vi "Best_Match.vi"(2 "Input String":string, 3 "String Options":string[](array[string])) -> (0 "Good Match":bool, 1 "index of element":i32)   [LabVIEW 2018]
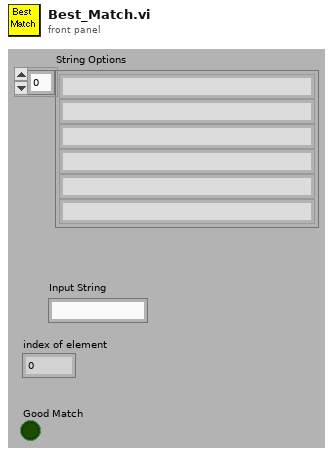
[diagram p1: front panel]
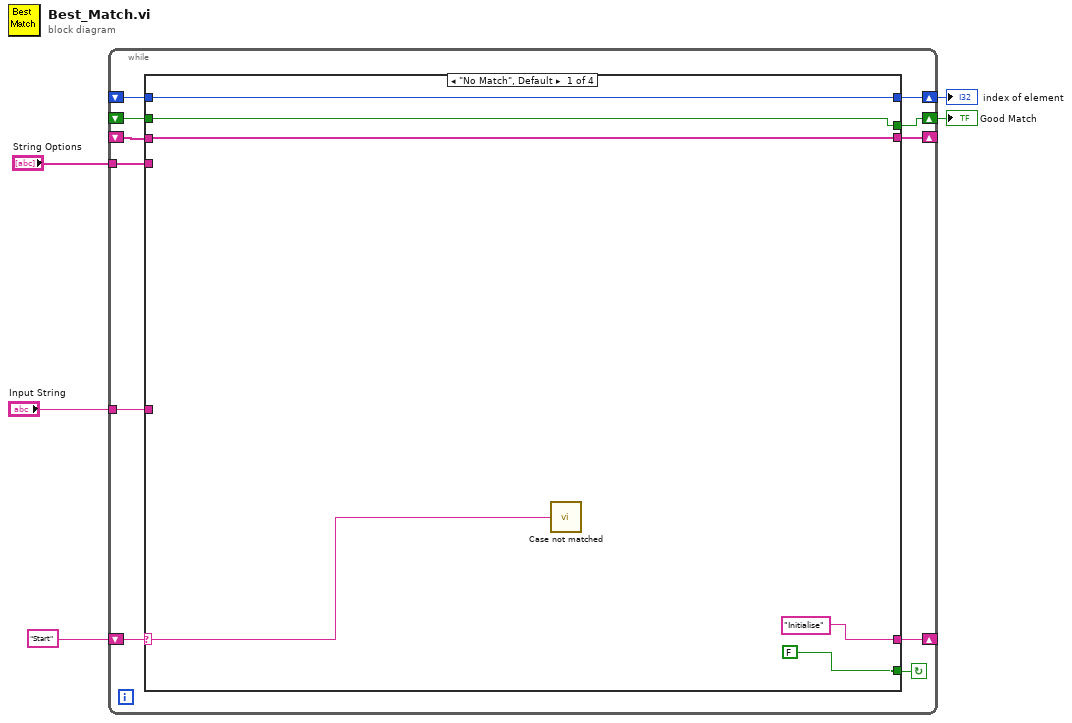
[diagram p0: block diagram]
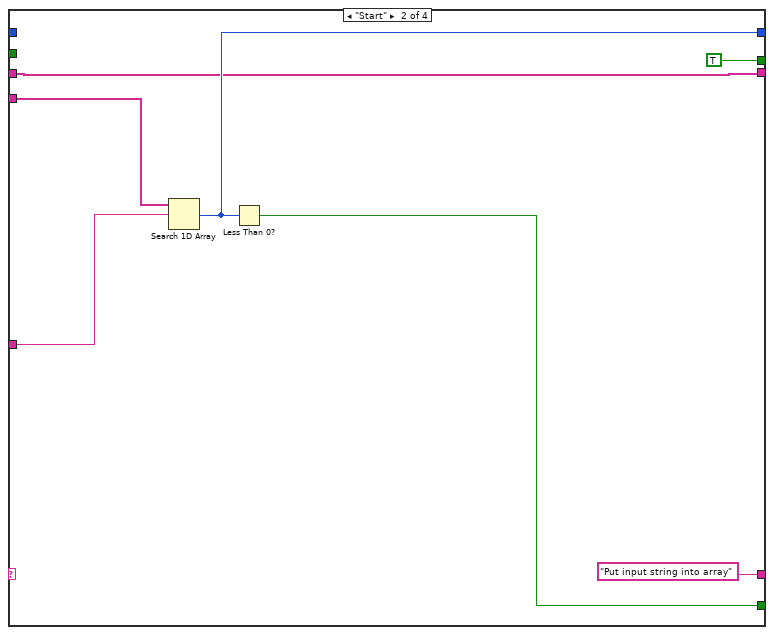
[diagram p2: hidden frame]
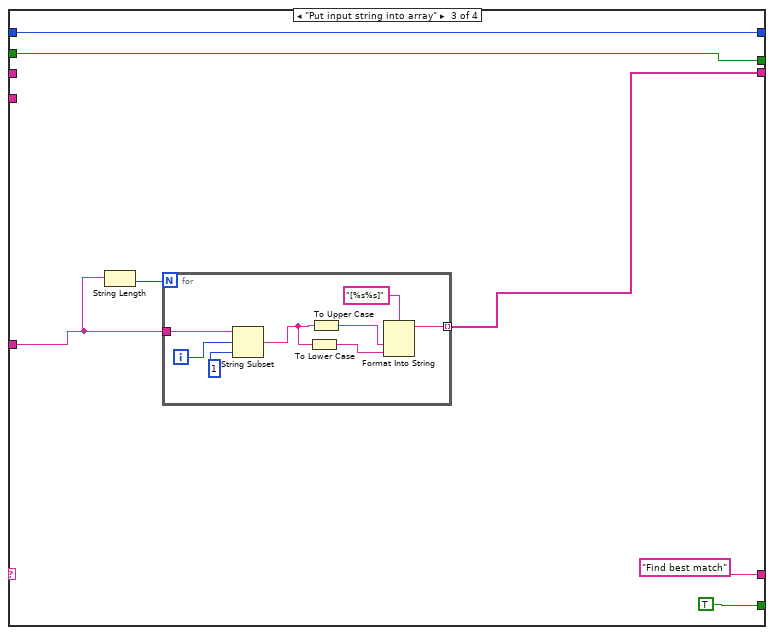
[diagram p3: hidden frame]
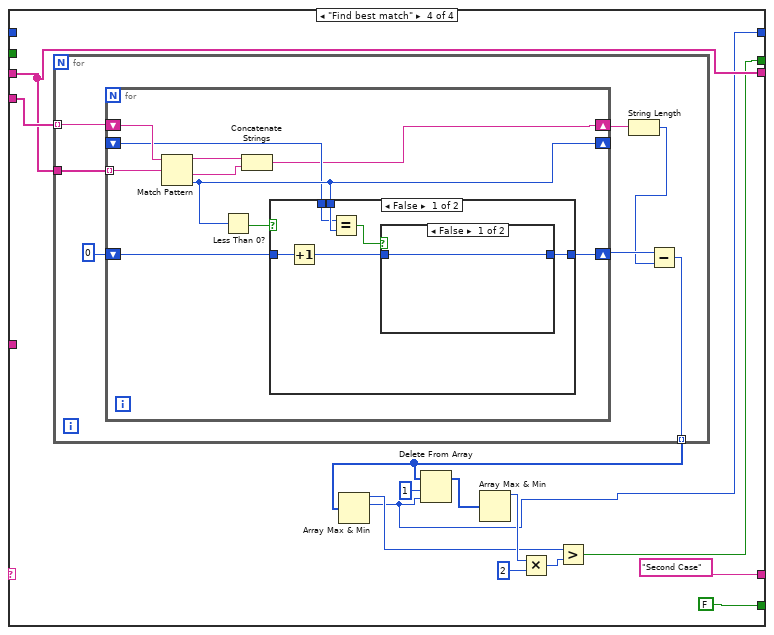
[diagram p4: hidden frame]
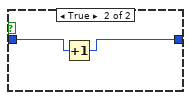
[diagram p5: hidden frame]
diagram:
  n1 = while {
    shift-left: "Start" -> [w14]
    shift-right: [w15] -> _
    tunnel: "String Options" -> [w13]
    tunnel: "Input String" -> [w12]
    shift-right: [w11] -> w2
    shift-left: _ -> [w9]
    shift-right: [w10] -> w1
    shift-left: _ -> [w8]
    shift-right: [w7] -> _
    shift-left: _ -> [w6]
    stop <- w16 continue-if-true
    n2 = case shown="\"No Match\", Default" w14 {
      selector: w14 -> [w17 _ _ _]
      tunnel: [FALSE w26 TRUE FALSE] -> w16
      tunnel: ["Initialise" "Put input string into array" "Find best match" "Second Case"] -> w15
      tunnel: w13 -> [_ w28 _ w55]
      tunnel: w12 -> [_ w27 w34 _]
      tunnel: [w20 w25 w31 w46] -> w11
      tunnel: [w19 TRUE w30 w45] -> w10
      tunnel: w9 -> [w20 _ w31 _]
      tunnel: w8 -> [w19 _ w30 _]
      tunnel: [w18 w24 w32 w54] -> w7
      tunnel: w6 -> [w18 w24 _ w54]
      frame "No Match", Default {
        n3 = call "Case not matched.vi"("Case Name not Matched"=w17) -> ()
      }
      frame "Start" {
        n4 = Search 1D Array(1D array=w28, element=w27) -> (index of element=w25:i32)  [unwired: 1 out]
        n5 = Less Than 0?(x=w25) -> (x < 0?=w26:bool)
      }
      frame "Put input string into array" {
        n6 = String Length(string=w34) -> (length=w33:i32)
        n7 = for {
          N: w33 -> [_]
          tunnel: w34 -> [w43]
          tunnel: [w37] -> w32 mode=indexing
          i -> [w38]
          n8 = String Subset(string=w43, offset (0)=w38, length (rest)=1 ("length (rest)")) -> (substring=w42:string)
          n9 = To Lower Case(string=w42) -> (all lower case string=w40:string)
          n10 = To Upper Case(1:w42) -> (0:w41:string)
          n11 = Format Into String(format string="[%s%s]", w41, w40) -> (resulting string=w37:string)  [unwired: 2 in, 1 out]
        }
      }
      frame "Find best match" {
        n12 = for {
          tunnel: w54 -> [w64]
          tunnel: w55 -> [w63] mode=indexing
          tunnel: [w58] -> w53 mode=indexing
          n13 = for {
            tunnel: w64 -> [w74] mode=indexing
            shift-right: [w65] -> w61
            shift-left: w63 -> [w73]
            shift-right: [w67] -> _
            shift-left: _ -> [w66]
            shift-right: [w69] -> w60
            shift-left: 0 -> [w68]
            n14 = Match Pattern(string=w73, regular expression=w74) -> (before substring=w72:string, after substring=w71:string, offset past match=w67:i32)  [unwired: 2 out]
            n15 = Less Than 0?(x=w67) -> (x < 0?=w70:bool)
            n16 = Concatenate Strings(w72, w71) -> (w65:string)
            n17 = case shown="False" w70 {
              tunnel: [w75 w84] -> w69
              tunnel: w68 -> [w80 w84]
              tunnel: w67 -> [w79 _]
              tunnel: w66 -> [w78 _]
              frame False {
                n18 = Increment(x=w80) -> (x+1=w76:i32)
                n19 = Equal?(x=w78, y=w79) -> (x = y?=w77:bool)
                n20 = case shown="False" w77 {
                  tunnel: w76 -> [w81 w83]
                  tunnel: [w81 w82] -> w75
                  frame False {
                  }
                  frame True {
                    n21 = Increment(x=w83) -> (x+1=w82:i32)
                  }
                }
              }
              frame True {
              }
            }
          }
          n22 = String Length(string=w61) -> (length=w59:i32)
          n23 = Subtract(x=w60, y=w59) -> (x-y=w58:i32)
        }
        n24 = Array Max & Min(array=w53) -> (max value=w47:i32, max index (indices)=w46:i32)  [unwired: 2 out]
        n25 = Delete From Array(array=w53, length=1, index=w46) -> (array with subset deleted=w51:i32[])  [unwired: 1 out]
        n26 = Array Max & Min(array=w51) -> (max value=w50:i32)  [unwired: 3 out]
        n27 = Multiply(x=w50, y=2) -> (x*y=w48:i32)
        n28 = Greater?(x=w47, y=w48) -> (0:w45:bool)
      }
    }
  }
  "index of element" <- w2
  "Good Match" <- w1
